vi "XIPIN_DDR3_SDRAM_(MIG)_1_1.vi"   [LabVIEW 2017]
doc: "Memory Interface Generator for generating DDR3 interfaces for Ultrascale Architecture\n------------------------------------\n<b>Need License</b> : No\n<b>Interface</b> : AXI4"
uses:
  <vilib>/rvi/XilinxIP/XIPIN_XNode/niFpgaXIPIN.xnode
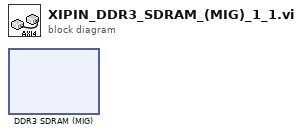
[diagram p0: block diagram]
diagram:
  n1 = xnode ("DDR3 SDRAM (MIG)")() -> ()
